vi "Anlage Spuelen.vi"(6 "Aktionen":T1, 11 "Spülen?":bool) -> (3 "Spülen?":bool)   [LabVIEW 2020, in "Allgemein.lvlib"]
uses:
  Allgemein.lvlib
  Anlage Spuelen Aktionen.ctl
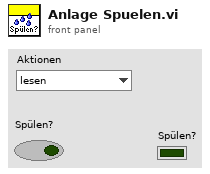
[diagram p1: front panel]
types:
  T1 = typedef "Allgemein.lvlib/Anlage Spuelen Aktionen.ctl" = enum16{"lesen", "spülen?"}
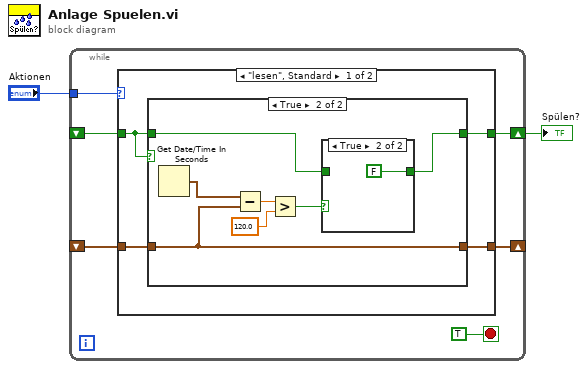
[diagram p0: block diagram]
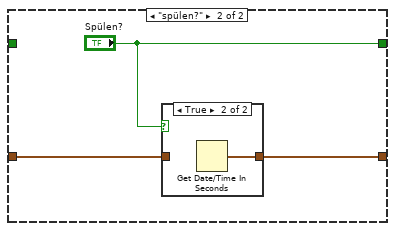
[diagram p4: hidden frame]
diagram:
  n1 = while {
    tunnel: "Aktionen" -> [w7]
    shift-right: [w6] -> w1
    shift-left: _ -> [w5]
    shift-right: [w4] -> _
    shift-left: _ -> [w3]
    stop <- TRUE stop-if-true
    n2 = case shown="\"lesen\", Standard" w7 {
      tunnel: [w9 "Spülen?"] -> w6
      tunnel: w5 -> [w10 _]
      tunnel: [w11 w25] -> w4
      tunnel: w3 -> [w12 w24]
      frame "lesen", Default {
        n3 = case shown="True" w10 {
          tunnel: w12 -> [w14 w17]
          tunnel: [w14 w17] -> w11
          tunnel: w10 -> [w13 w16]
          tunnel: [w13 w15] -> w9
          frame False {
          }
          frame True {
            n4 = Get Date/Time In Seconds() -> (seconds since 1Jan1904=w21:timestamp)
            n5 = Subtract(x=w21, y=w17) -> (x-y=w20:dbl)
            n6 = Greater?(x=w20, y=120.0) -> (0:w18:bool)
            n7 = case shown="True" w18 {
              tunnel: w16 -> [w22 _]
              tunnel: [w22 FALSE ("Spülen?")] -> w15
              frame False {
              }
              frame True {
              }
            }
          }
        }
      }
      frame "spülen?" {
        n8 = case shown="True" "Spülen?" {
          tunnel: [w27 w28] -> w25
          tunnel: w24 -> [w27 _]
          frame False {
          }
          frame True {
            n9 = Get Date/Time In Seconds() -> (seconds since 1Jan1904=w28:timestamp)
          }
        }
      }
    }
  }
  "Spülen?" <- w1
